vi "Distance Operation.vi"(11 "мм":dbl=3.0) -> (3 "ослабление":dbl)   [LabVIEW 2019]
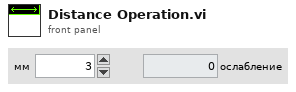
[diagram p1: front panel]
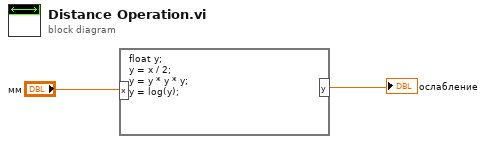
[diagram p0: block diagram]
diagram:
  n1 = formula code="float y;\ny = x / 2;\ny = y * y * y;\ny = log(y);"("x"="мм") -> ("y"=→"ослабление":dbl)
